vi "Get All Component Settings.vi"(8 "error in (no error)":errorcluster, 11 "Runtime Configuration in":refnum<class "Core Configuration.lvclass">) -> (0 "error out":errorcluster, 2 "component settings":T1[](array[typedef]), 3 "Runtime Configuration out":refnum<class "Core Configuration.lvclass">)   [LabVIEW 2020, in "DSF Core.lvlib" / "Core Configuration.lvclass"]
uses:
  Core Configuration.lvclass
  Typedefs/DSF Settings Info.ctl
  Core Configuration.lvclass/Core Configuration.ctl
  DSF Core.lvlib
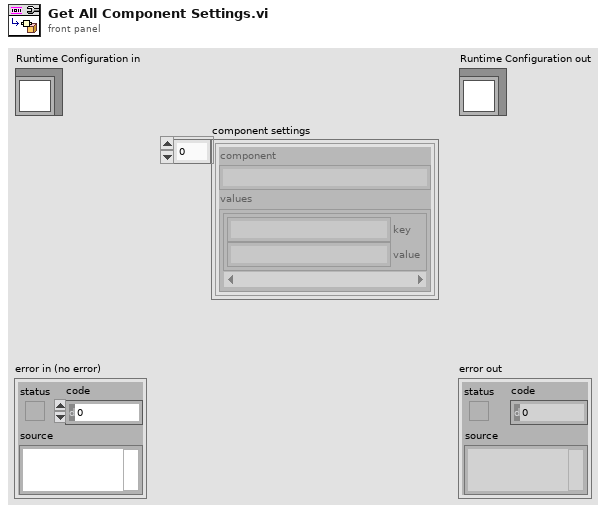
[diagram p1: front panel]
types:
  T1 = typedef "DSF Core.lvlib/DSF Settings Info.ctl" = cluster{"component":string, "values":cluster{"key":string, "value":string}[]}
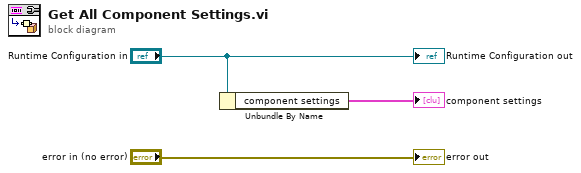
[diagram p0: block diagram]
diagram:
  n1 = Unbundle By Name("Runtime Configuration in") -> ("component settings"=→"component settings":T1[])
  "error out" <- "error in (no error)"
  "Runtime Configuration out" <- "Runtime Configuration in"
